vi "TestSCAN.vi"(8 "errin":errorcluster) -> (0 "error out":errorcluster, 2 "COM VUS":refnum<visa-resource-name>[](array[refnum]), 3 "Retour IDN":string[](array[string]))   [LabVIEW 2020]
doc: "Ce VI te sniff tout les équipement VISA qu'il détect et t'en fait une liste"
uses:
  <vilib>/Instr/_visa.llb/VISA Find Search Mode.ctl
  <vilib>/MakerHub/LINX/Public/Utilities/Open Serial.vi
  <vilib>/MakerHub/LINX/LMH-LINX.lvlib
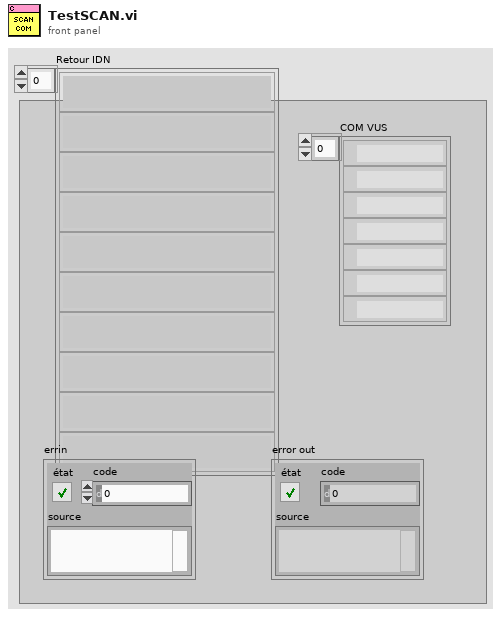
[diagram p1: front panel]
types:
  T1 = typedef "VISA Find Search Mode.ctl" = u32
  T2 = typedef "LMH-LINX.lvlib/LINX Ref.ctl" = cluster{"IO":T3, "Interface":T4, "LINX Device Config":T5}
  T3 = typedef "LMH-LINX.lvlib/Platform.ctl" = enum16{"Remote", "Local"}
  T4 = typedef "LMH-LINX.lvlib/Interface.ctl" = enum16{"Serial", "TCP"}
  T5 = typedef "LMH-LINX.lvlib/Device.lvlib/LINX Device Config.ctl" = cluster{"Interface":T4, "COM Port":refnum<visa-resource-name>, "TCP Configuration":T6, "Device Family":u8, "Device ID":u8, "Device Name":string, "TCP Ref":refnum<k5>, "Channels":T7}
  T6 = typedef "LMH-LINX.lvlib/Device.lvlib/TCP Config.ctl" = cluster{"IP Address":string, "Port":u16}
  T7 = typedef "LMH-LINX.lvlib/Channels.ctl" = cluster{"DI":u8[], "DO":u8[], "AI":u8[], "AO":u8[], "PWM":u8[], "QE":u8[], "UART":u8[], "I2C 2":u8[], "SPI":u8[], "CAN":u8[], "Servo":u8[], "AI Ref (V)":dbl, "AI Resolution (Bits)":u8, "AO Ref (V)":dbl, "AO Resolution (Bits)":u8}
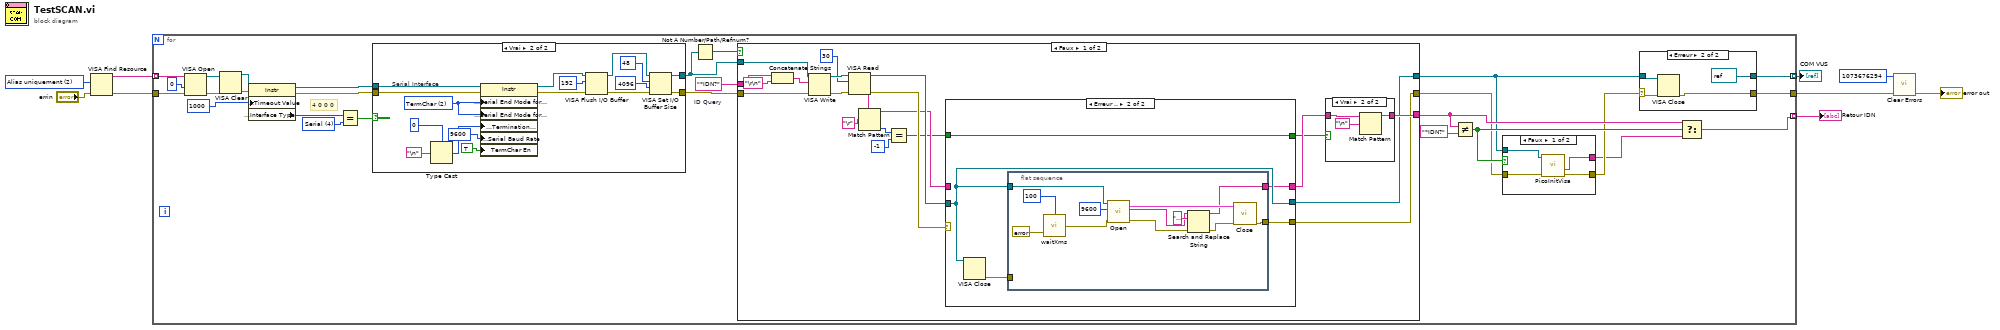
[diagram p0: block diagram]
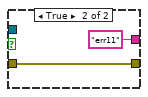
[diagram p2: hidden frame]
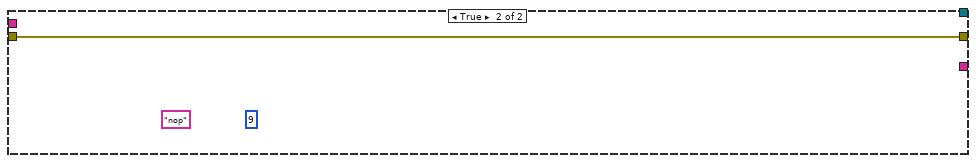
[diagram p5: hidden frame]
diagram:
  w5 = T1 2 items=["Noms canoniques uniquement"=0, "Alias uniquement"=2, "Inclure les alias correspondants"=3, "Inclure tous les alias"=4] ("Search Mode")
  n1 = VISA Find Resource(8:"errin", 10:w5) -> (0:w4:errorcluster, 3:w9:string[])  [unwired: 1 in, 1 out]
  n2 = for {
    tunnel: w9 -> [w31] mode=indexing
    tunnel: [w17] -> w8 mode=indexing
    tunnel: [w26] -> w6 mode=indexing
    tunnel: w4 -> [w30]
    tunnel: [w27] -> w3
    w28 = "*IDN?"  # ID Query
    w25 = u16 4 items=["GPIB"=1, "VXI"=2, "GPIB-VXI"=3, "Serial"=4, "PXI"=5, "TCPIP"=6, "USB"=7] ("Interface Information:Interface Type")
    # "4 0 0 0"
    n3 = VISA Open(access mode=u32 0, error in (no error)=w30, VISA resource name=w31) -> (VISA resource name=w13:refnum<visa-resource-name>, error out=w11:errorcluster)  [unwired: 2 in]
    n4 = VISA Clear(VISA resource name=w13, error in (no error)=w11) -> (VISA resource name out=w12:refnum<visa-resource-name>, error out=w10:errorcluster)
    n5 = property class="Instr"(reference=w12, error in=w10, "General Settings:Timeout Value"=u32 1000) -> (reference out=w34:refnum<visa-resource-name>, error out=w33:errorcluster, "Interface Information:Interface Type"=w16:u16)
    n6 = Equal?(x=w16, y=w25) -> (x = y?=w14:bool)
    n7 = case shown="Vrai" w14 {
      tunnel: [w90 w105] -> w35
      tunnel: [w91 w102] -> w15
      tunnel: w34 -> [w90 w107]
      tunnel: w33 -> [w91 w108]
      frame False {
        # "EDIT: Remove interfaces not supported by your instrument."
        # "GPIB, TCP/IP, and USB Interface"
      }
      frame True {
        w95 = u16 2 items=["None", "LastBit", "TermChar"] ("Serial Settings:Serial End Mode for Reads")
        # "Serial Interface"
        n8 = Type Cast(type=u8 0, x="\n" ("Line Feed Constant")) -> (*(type *) &x=w94:u8)
        n9 = property class="Instr"(reference=w107, error in=w108, "Serial Settings:Serial End Mode for Reads"=w95, "Serial Settings:Serial End Mode for Writes"=w95, "Message Based Settings:Termination Character"=w94, "Serial Settings:Serial Baud Rate"=u32 9600 ("Serial Settings:Baud Rate"), "TermChar En"=TRUE ("Message Based Settings:Termination Character Enable")) -> (reference out=w101:refnum<visa-resource-name>, error out=w104:errorcluster)
        n10 = VISA Flush I/O Buffer(VISA resource name=w101, mask (16)=u16 192, error in (no error)=w104) -> (VISA resource name out=w106:refnum<visa-resource-name>, error out=w103:errorcluster)
        n11 = VISA Set I/O Buffer Size(VISA resource name=w106, mask (16)=u16 48, size (4096)=u32 4096 ("size (0)"), error in (no error)=w103) -> (VISA resource name out=w105:refnum<visa-resource-name>, error out=w102:errorcluster)
      }
    }
    n12 = Not A Number/Path/Refnum?(number/path/refnum=w35) -> (NaN/Path/Refnum?=w29:bool)
    n13 = case shown="Faux" w29 {
      tunnel: [w47 _] -> w19
      tunnel: [w49 w89] -> w21
      tunnel: [w57 _] -> w23
      tunnel: w35 -> [w50 _]
      tunnel: w28 -> [w56 _]
      tunnel: w15 -> [w54 w89]
      frame False {
        n14 = Concatenate Strings(w56, "\r\n") -> (w60:string)
        n15 = VISA Write(VISA resource name=w50, write buffer=w60, error in (no error)=w54) -> (VISA resource name out=w63:refnum<visa-resource-name>, error out=w62:errorcluster)  [unwired: 1 out]
        n16 = VISA Read(VISA resource name=w63, byte count=u32 30 ("nombre d'octets"), error in (no error)=w62) -> (VISA resource name out=w48:refnum<visa-resource-name>, read buffer=w53:string, error out=w51:errorcluster)  [unwired: 1 out]
        n17 = Match Pattern(string=w53, regular expression="\r") -> (before substring=w46:string, offset past match=w52:i32)  [unwired: 1 in, 2 out]
        n18 = Equal?(x=w52, y=-1) -> (x = y?=w44:bool)
        n19 = case shown="Erreur .." w51 {
          selector: w51 -> [w67 _]
          tunnel: w48 -> [w66 w70]
          tunnel: [w67 w72] -> w49
          tunnel: [w66 w70] -> w47
          tunnel: w46 -> [w65 _]
          tunnel: [w65 w68] -> w45
          tunnel: w44 -> [w64 w69]
          tunnel: [w64 w69] -> w43
          frame No Error {
          }
          frame Error {
            n20 = VISA Close(VISA resource name=w70) -> (error out=w71:errorcluster)  [unwired: 1 in]
            n21 = flat-sequence {
              tunnel: [w83] -> w72
              tunnel: w71 -> [_]
              tunnel: w70 -> [w78]
              tunnel: [w75] -> w68
              frame #0 {
                n22 = call <vilib>:"waitXms.vi"("attente (ms)"=u32 100, "errin"=errorcluster {"status"=FALSE, "code"=0, "source"=""} ("Error In")) -> ("errout"=w80:errorcluster)  [unwired: 13 in]
                n23 = call-poly <vilib>:"Open.vi"("Error In"=w80, "Baud Rate Override"=u32 9600, "Serial Port"=w78) -> ("Error Out"=w74:errorcluster, "Device Name"=w76:string, "LINX Resource"=w84:T2)  [unwired: 6 in]
                n24 = Search and Replace String ("Rechercher et remplacer une chaîne")(input string=w76, search string="\u0000" ("chaîne recherchée"), error in=w74) -> (result string=w75:string, error out=w73:errorcluster)  [unwired: 5 in, 2 out]
                n25 = call <vilib>:"Close.vi"("Error In"=w73, "LINX Resource"=w84) -> ("Error Out"=w83:errorcluster)  [unwired: 9 in]
              }
            }
          }
        }
        n26 = case shown="Vrai" w43 {
          tunnel: w45 -> [w85 w87]
          tunnel: [w85 w86] -> w57
          frame False {
          }
          frame True {
            n27 = Match Pattern(string=w87, regular expression="\n") -> (before substring=w86:string)  [unwired: 1 in, 3 out]
          }
        }
      }
      frame True {
        (unwired) 9 ("offset past match")
        (unwired) "nop" ("read buffer")
      }
    }
    n28 = Not Equal?(x=w23, y="*IDN?") -> (x != y?=w22:bool)
    n29 = case shown="Faux" w22 {
      tunnel: w21 -> [w40 w42]
      tunnel: [w39 w42] -> w20
      tunnel: w19 -> [w38 _]
      tunnel: [w37 "err11" ("data out")] -> w18
      frame False {
        n30 = call "PicoInitVisa.vi"("errin"=w40, "visain"=w38) -> ("sortie d'erreur"=w39:errorcluster, "buffer de lecture 2"=w37:string)  [unwired: 6 in, 2 out]
      }
      frame True {
      }
    }
    n31 = case shown="Erreur" w20 {
      selector: w20 -> [w109 w113]
      tunnel: w19 -> [w110 w112]
      tunnel: [w110 refnum<visa-resource-name> refnum ("VISA resource name out")] -> w26
      tunnel: [w109 w111] -> w27
      frame No Error {
      }
      frame Error {
        n32 = VISA Close(VISA resource name=w112, error in (no error)=w113) -> (error out=w111:errorcluster)
      }
    }
    n33 = Select(t=w23, s=w22, f=w18) -> (s? t:f=w17:string)
  }
  "Retour IDN" <- w8
  "COM VUS" <- w6
  n34 = call <vilib>:"Clear Errors.vi"("error in (no error)"=w3, "specific error code to clear (0: all)"=1073676294) -> ("error out"=→"error out":errorcluster)  [unwired: 4 in, 1 out]
